vi "CheckScreenShot (SubVI).vi"(2 "VI reference":refnum<vi>) -> ()   [LabVIEW 8.6]
uses:
  <vilib>/picture/picture.llb/Draw True-Color Pixmap.vi
panel:
  out "ScreenShot":picture
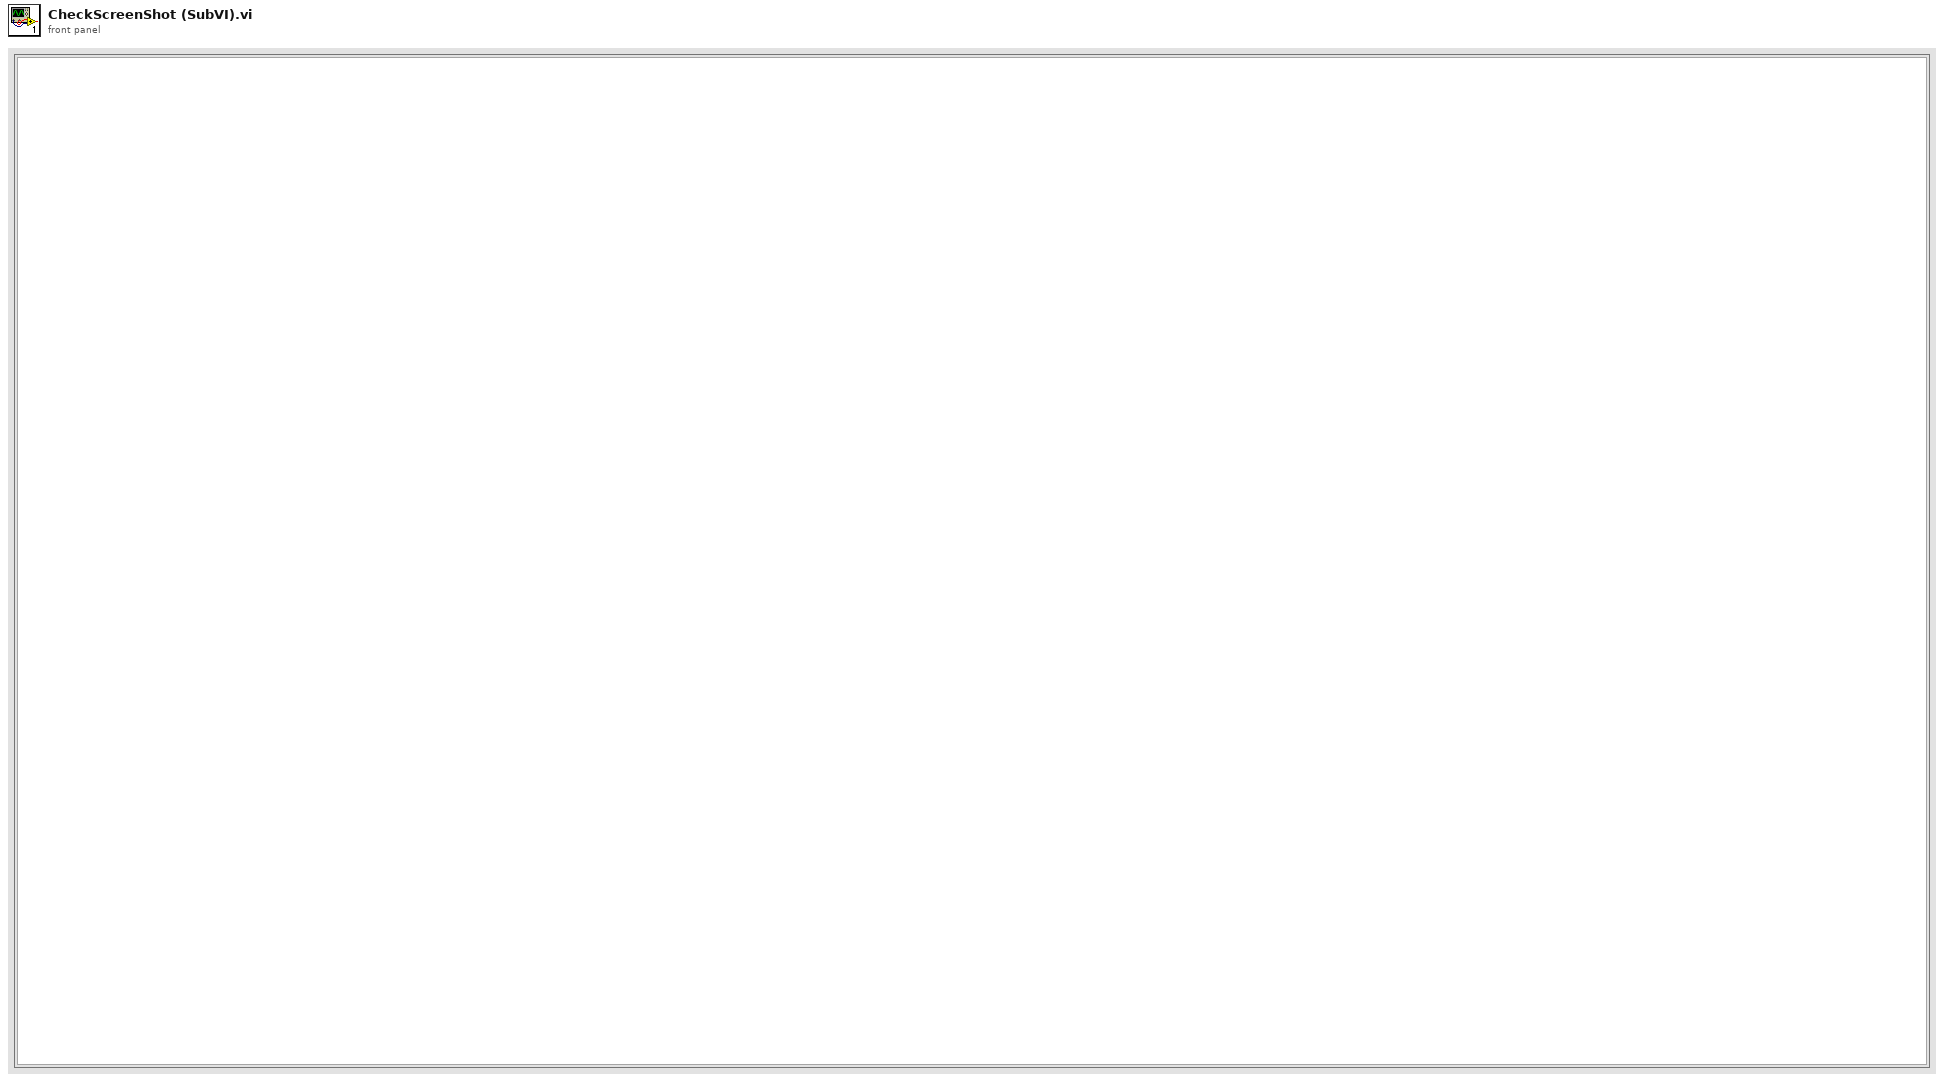
[diagram p1: front panel]
types:
  T1 = typedef "imagedata.ctl" = cluster{"image type":i32, "image depth":i32, "image":u8[], "mask":u8[], "colors":u32[], "Rectangle":cluster{"left":i16, "top":i16, "right":i16, "bottom":i16}}
  T2 = typedef "LVRectTypeDef.ctl" = cluster{"Left":i16, "Top":i16, "Right":i16, "Bottom":i16}
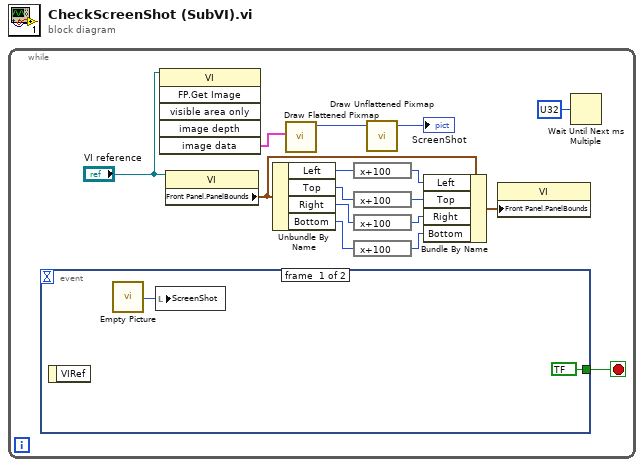
[diagram p0: block diagram]
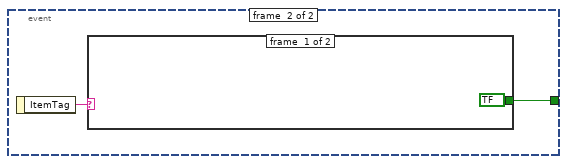
[diagram p2: hidden frame]
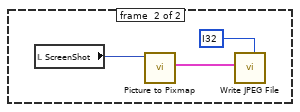
[diagram p3: hidden frame]
diagram:
  n1 = while {
    stop <- w2 stop-if-true
    n2 = event shown="[1] Menu Selection (User)" {
      selector: _ -> [_ _]
      dyn-events: _ -> [_ _]
      timeout: _ -> [_ _]
      tunnel: [bool ? w19] -> w2
      event #0 {
        n3 = event-data() -> ()  [unwired: 1 in, 1 out]
        n4 = call "Empty Picture"() -> ("empty picture"=w18:picture)
        n5 = local write "ScreenShot"(w18) -> ()
      }
      event #1 {
        n6 = event-data() -> ("ItemTag"=w20:string)  [unwired: 1 in]
        n7 = case shown="\"Сохранить как ...\", Default" w20 {
          tunnel: [bool ? _] -> w19
          frame #0 {
          }
          frame #1 {
            n8 = local read "ScreenShot"() -> (w24:picture)
            n9 = call <vilib>:"Picture to Pixmap.vi"("picture"=w24) -> ("image data"=w22:T1)  [unwired: 9 in, 1 out]
            n10 = call <vilib>:"Write JPEG File.vi"("quality (80)"=i32 ?, "image data"=w22) -> ()  [unwired: 2 in, 8 out]
          }
        }
      }
    }
    n11 = invoke class="VI" method="FP.Get Image"(reference="VI reference") -> ("image data"=w14:T1)  [unwired: 5 in, 5 out]
    n12 = property class="VI"(reference="VI reference") -> ("Front Panel.PanelBounds"=w8:T2)  [unwired: 1 in, 2 out]
    n13 = Unbundle By Name(w8) -> ("Left"=w12:i16, "Top"=w11:i16, "Right"=w10:i16, "Bottom"=w9:i16)
    n14 = call <vilib>:"Draw Flattened Pixmap.vi"("image data"=w14) -> ("new picture"=w13:picture)  [unwired: 8 in]
    n15 = expression code="x+100"(w12) -> (w7:i16)
    n16 = expression code="x+100"(w11) -> (w6:i16)
    n17 = expression code="x+100"(w10) -> (w5:i16)
    n18 = expression code="x+100"(w9) -> (w4:i16)
    n19 = call-poly <vilib>:"Draw Unflattened Pixmap.vi"("picture"=w13) -> ("new picture"=→"ScreenShot":picture)  [unwired: 8 in]
    n20 = Bundle By Name(cluster=w8, "Left"=w7, "Top"=w6, "Right"=w5, "Bottom"=w4) -> (w3:T2)
    n21 = property class="VI"("Front Panel.PanelBounds"=w3) -> ()  [unwired: 2 in, 2 out]
    n22 = Wait Until Next ms Multiple(millisecond multiple=u32 ?) -> ()  [unwired: 1 out]
  }
